vi "getDelay.vi"(8 "error in (no error)":errorcluster, 11 "Instrument.Delay in":refnum<class "Instrument.DelayLine.lvclass">) -> (0 "error out":errorcluster, 2 "Delay (ps)":dbl, 3 "Instrument.Delay out":refnum<class "Instrument.DelayLine.lvclass">, 4 "Finished?":bool)   [LabVIEW 2019, in "Instrument.DelayLine.lvclass"]
uses:
  Instrument.DelayLine.lvclass
  C:/Users/patrick/Documents/GitHub/Instrument-Framework/lvsrc/Instrument/Instrument.lvclass
  Instrument/Instrument.lvclass/Instrument.ctl
  fe7b943a-5057-46fe-8def-e8bcae168474.vi
  fe7b943a-5057-46fe-8def-e8bcae168474.vi/67f80931-ad2b-4374-94b2-fc56382d5274.vi
  fe7b943a-5057-46fe-8def-e8bcae168474.vi/b18bab1e-f066-427a-be92-0a2222c7cc8f.vi
  Instrument/Private/Get Client Type.vi
  fe7b943a-5057-46fe-8def-e8bcae168474.vi/67f80931-ad2b-4374-94b2-fc56382d5274.vi/b8453210-f7d6-42a5-82db-e25154306242.vi
  fe7b943a-5057-46fe-8def-e8bcae168474.vi/67f80931-ad2b-4374-94b2-fc56382d5274.vi/de227407-9258-4864-9c9d-b7a934ec5720.vi
  Instrument/Private/Set Dependencies.vi
  fe7b943a-5057-46fe-8def-e8bcae168474.vi/b18bab1e-f066-427a-be92-0a2222c7cc8f.vi/0214074c-0a75-4a3f-919e-1a8617975d23.vi
  fe7b943a-5057-46fe-8def-e8bcae168474.vi/b18bab1e-f066-427a-be92-0a2222c7cc8f.vi/cac9e569-e1a0-4b8d-b8ee-093fd18ced25.vi
  fe7b943a-5057-46fe-8def-e8bcae168474.vi/b18bab1e-f066-427a-be92-0a2222c7cc8f.vi/c6c82c24-019e-4793-9fd4-e3f82ae547e8.vi
  fe7b943a-5057-46fe-8def-e8bcae168474.vi/67f80931-ad2b-4374-94b2-fc56382d5274.vi/de227407-9258-4864-9c9d-b7a934ec5720.vi/52d27cf0-dc64-4d81-8afd-eef84b8e7066.vi
  fe7b943a-5057-46fe-8def-e8bcae168474.vi/67f80931-ad2b-4374-94b2-fc56382d5274.vi/de227407-9258-4864-9c9d-b7a934ec5720.vi/69c6730f-c91f-4154-b5ea-7805a9d3b593.vi
  fe7b943a-5057-46fe-8def-e8bcae168474.vi/b18bab1e-f066-427a-be92-0a2222c7cc8f.vi/cac9e569-e1a0-4b8d-b8ee-093fd18ced25.vi/45542101-dcd5-4950-9a4d-26e07ddffa72.vi
  fe7b943a-5057-46fe-8def-e8bcae168474.vi/b18bab1e-f066-427a-be92-0a2222c7cc8f.vi/cac9e569-e1a0-4b8d-b8ee-093fd18ced25.vi/6719eb20-3374-4966-be94-04ae4273fee9.vi
  fe7b943a-5057-46fe-8def-e8bcae168474.vi/b18bab1e-f066-427a-be92-0a2222c7cc8f.vi/c6c82c24-019e-4793-9fd4-e3f82ae547e8.vi/ac6e9945-bb17-4988-8e84-ab00022367f0.vi
  fe7b943a-5057-46fe-8def-e8bcae168474.vi/b18bab1e-f066-427a-be92-0a2222c7cc8f.vi/c6c82c24-019e-4793-9fd4-e3f82ae547e8.vi/60affa43-c283-4da7-b928-d04cbfce3b37.vi
  Instrument/Private/Get RC Connection Status.vi
  Instrument/Private/Get Dependencies.vi
  <userlib>/LevyLab/RemoteControl/API/Send and Receive.vi
  <vilib>/Utility/Data Type/Get Type Information.vi
  <vilib>/JDP Science/JSONtext/JSON text to Variant.vi
  Instrument/API/Instrument.GetPublicEvents.vi
  <vilib>/JDP Science/JSONtext/Variant to JSON Text.vi
  <vilib>/National Instruments/GUID Generator/Guid Generator.vi
  Instrument/API/Instrument.sendMessageToProcess.vi
  Instrument/Private/Instrument.MessageFromProcess.EventStructure.vi
  <vilib>/JDP Science/JSONtext/LVClass Serializer/JSONtext LVClass Serializer.lvclass
  Instrument/Instrument.lvclass
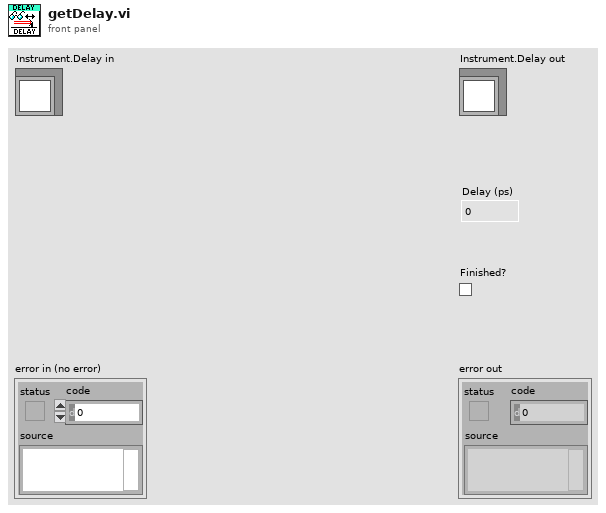
[diagram p1: front panel]
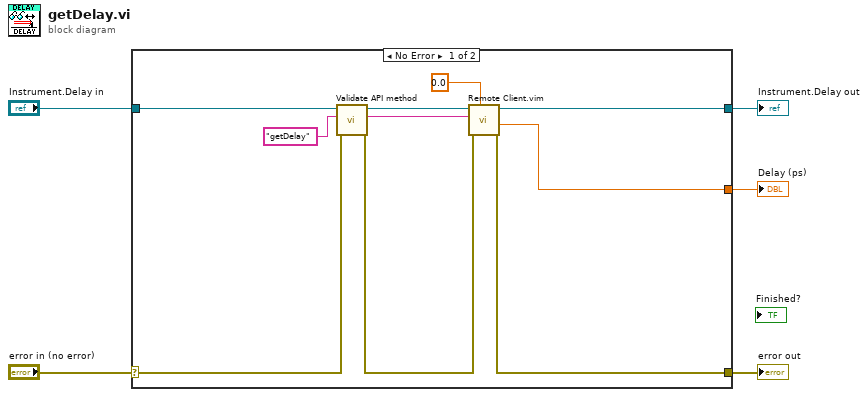
[diagram p0: block diagram]
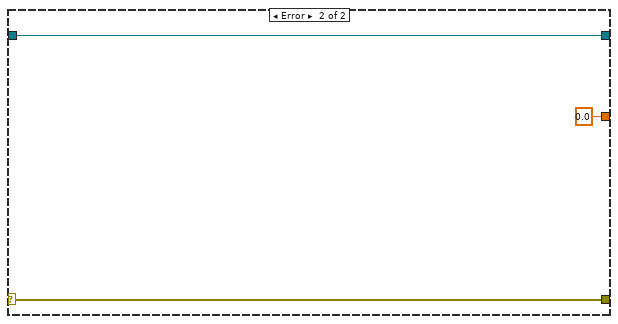
[diagram p2: hidden frame]
diagram:
  n1 = case shown="No Error" "error in (no error)" {
    selector: "error in (no error)" -> [w10 w18]
    tunnel: [w8 w18] -> w4
    tunnel: [w7 w17] -> w2
    tunnel: "Instrument.Delay in" -> [w11 w17]
    tunnel: [w6 0.0 ("Data out")] -> w1
    frame No Error {
      n2 = call "Validate API method.vi"("error in (no error)"=w10, "command in"="getDelay" ("error message (\"\")"), "Instrument in"=w11) -> ("error out"=w9:errorcluster, "command out"=w13:string, "Instrument out"=w12:refnum<class "Instrument.DelayLine.lvclass">)  [unwired: 6 in]
      n3 = call "Remote Client.vim"("Data Out type"=0.0, "error in (no error)"=w9, "method"=w13, "Instrument in"=w12) -> ("error out"=w8:errorcluster, "Data out"=w6:dbl, "Instrument out"=w7:refnum<class "Instrument.DelayLine.lvclass">)  [unwired: 4 in, 1 out]
    }
    frame Error {
    }
  }
  "error out" <- w4
  "Instrument.Delay out" <- w2
  "Delay (ps)" <- w1
